vi "myRIO_BRig_RT_dataLick_time__atLick.vi"() -> (2 "output_time__atLick":i32)   [LabVIEW 2014]
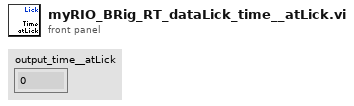
[diagram p1: front panel]
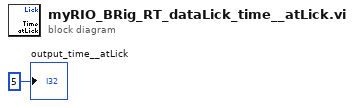
[diagram p0: block diagram]
diagram:
  "output_time__atLick" <- 5 ("output_iBlock")
